vi "Set Device Data Characteristics.vi"(8 "error in (no error)":errorcluster, 10 "Data Characteristics":T1={"Word Length"=8, "Stop Bits"=0, "Parity"=0} {"Parity" items=["FT_PARITY_NONE", "FT_PARITY_ODD", "FT_PARITY_EVEN", "FT_PARITY_MARK", "FT_PARITY_SPACE"]; "Stop Bits" items=["FT_STOP_BITS_1"=0, "FT_STOP_BITS_2"=2]; "Word Length" items=["FT_BITS_7"=7, "FT_BITS_8"=8]}, 11 "Handle":u64) -> (0 "error out":errorcluster, 3 "Handle out":u64)   [LabVIEW 2019, in "D2XX-lv.lvlib"]
doc: "This function sets the data characteristics for an open device."
uses:
  D2XX-lv.lvlib
  <instrlib>/_D2XX/D2XX/D2XX.lvlib
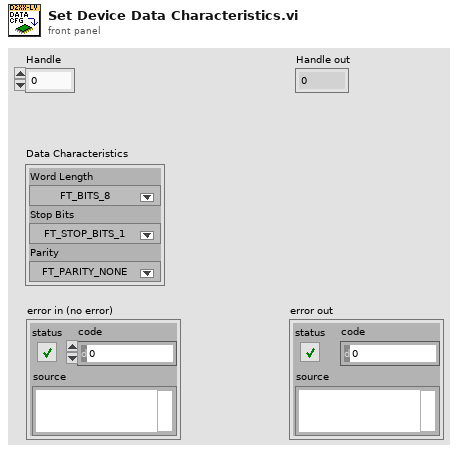
[diagram p1: front panel]
types:
  T1 = cluster{"Word Length":u8, "Stop Bits":u8, "Parity":u8}
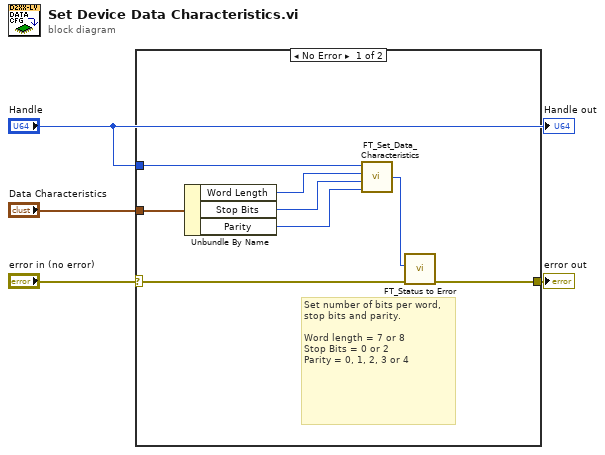
[diagram p0: block diagram]
diagram:
  n1 = case shown="No Error" "error in (no error)" {
    selector: "error in (no error)" -> [w12 w13]
    tunnel: [w10 w13] -> w3
    tunnel: "Handle" -> [w9 _]
    tunnel: "Data Characteristics" -> [w8 _]
    frame No Error {
      # "Set number of bits per word, stop bits and parity.\n\nWord length = 7 or 8\nStop Bits = 0 or 2\nParity = 0, 1, 2, 3 or 4"
      n2 = Unbundle By Name(w8) -> ("Word Length"=w7:u8, "Stop Bits"=w6:u8, "Parity"=w5:u8)
      n3 = call <instrlib>:"FT_Set_Data_Characteristics.vi"("Parity"=w5, "Stop Bits"=w6, "Word Length"=w7, "Handle"=w9) -> ("FT_Status"=w11:u32)
      n4 = call "FT_Status to Error.vi"("error in (no error)"=w12, "FT_Status"=w11) -> ("error out"=w10:errorcluster)  [unwired: 9 in]
    }
    frame Error {
    }
  }
  "error out" <- w3
  "Handle out" <- "Handle"
